vi "Shooter Solenoid Refnums fg.vi"(0 "Menu":T8, 1 "Shooter Solenoid DevRef":T4={"DevStatus"={"status"=FALSE, "code"=0, "source"=""}, "Solenoid Module"=enum."Solenoid Module 1", "Forward Solenoid Channel"=enum."Invalid", "Reverse Solenoid Channel"=enum."Invalid"}, 2 "Latch Solenoid DevRef":T4={"DevStatus"={"status"=FALSE, "code"=0, "source"=""}, "Solenoid Module"=enum."Solenoid Module 1", "Forward Solenoid Channel"=enum."Invalid", "Reverse Solenoid Channel"=enum."Invalid"}, 3 "Right Up DevRef":T1={"DevStatus"={"status"=FALSE, "code"=0, "source"=""}, "DIO Channel"=enum."Invalid", "Digital Module"=enum."Digital Module 1"}, 4 "Right Down DevRef":T1={"DevStatus"={"status"=FALSE, "code"=0, "source"=""}, "DIO Channel"=enum."Invalid", "Digital Module"=enum."Digital Module 1"}, 5 "Hold Sensor DevRef":T1={"DevStatus"={"status"=FALSE, "code"=0, "source"=""}, "DIO Channel"=enum."Invalid", "Digital Module"=enum."Digital Module 1"}, 8 "DevRef to Get":T7(ring)) -> (14 "Selected Solenoid":T4={"DevStatus"={"status"=FALSE, "code"=0, "source"=""}, "Solenoid Module"=enum."Solenoid Module 1", "Forward Solenoid Channel"=enum."Invalid", "Reverse Solenoid Channel"=enum."Invalid"}, 15 "Selected Sensor":T1)   [LabVIEW 2013]
uses:
  <vilib>/Rock Robotics/WPI/Solenoid/WPI_SolenoidDevRef.ctl
  <vilib>/Rock Robotics/SystemInterfaces/Typedef/FPGA_TypedefSolenoidModule.ctl
  <vilib>/Rock Robotics/WPI/Solenoid/WPI_SolenoidChannel.ctl
  <vilib>/Rock Robotics/WPI/DigitalInput/WPI_DigitalInputDevRef.ctl
  <vilib>/Rock Robotics/SystemInterfaces/DIO/FPGA_DIOChannel.ctl
  <vilib>/Rock Robotics/SystemInterfaces/Typedef/FPGA_TypedefDigitalModule.ctl
  typedefs/fg_typedef.ctl
panel:
  out "Hold Sensor DevRef":T1
  out "Right Down DevRef":T1
  out "Right Up DevRef":T1
  out "Latch Solenoid DevRef":T4={"DevStatus"={"status"=FALSE, "code"=0, "source"=""}, "Solenoid Module"=enum."Solenoid Module 1", "Forward Solenoid Channel"=enum."Invalid", "Reverse Solenoid Channel"=enum."Invalid"}
  out "Shooter Solenoid DevRef":T4={"DevStatus"={"status"=FALSE, "code"=0, "source"=""}, "Solenoid Module"=enum."Solenoid Module 1", "Forward Solenoid Channel"=enum."Invalid", "Reverse Solenoid Channel"=enum."Invalid"}
  # "A Functional Global that stores refnums for \ncommonly used devices \nso as to not need to get them repeatedly"
  # "Option to Select Also..."
  # "it is only set once"
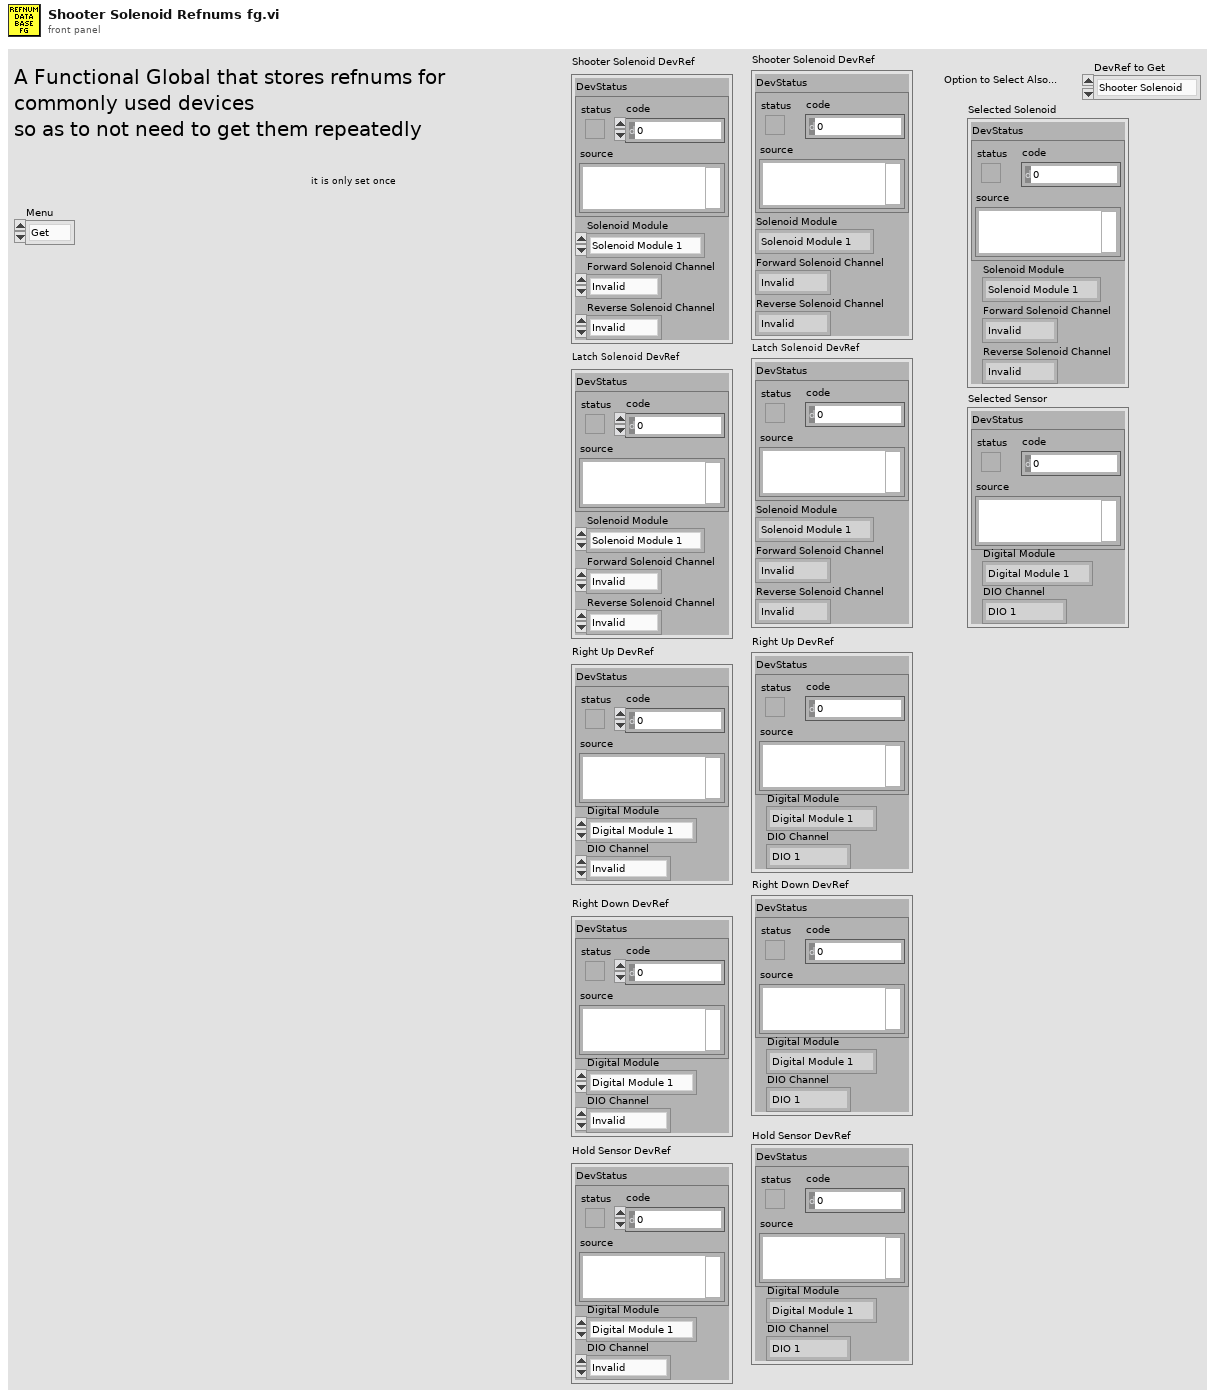
[diagram p1: front panel]
types:
  T1 = typedef "WPI_DigitalInputDevRef.ctl" = cluster{"DevStatus":errorcluster, "DIO Channel":T2, "Digital Module":T3}
  T2 = typedef "FPGA_DIOChannel.ctl" = enum8{"DIO 1", "DIO 2", "DIO 3", "DIO 4", "DIO 5", "DIO 6", "DIO 7", "DIO 8", "DIO 9", "DIO 10", "DIO 11", "DIO 12", "DIO 13", "DIO 14", "Invalid"}
  T3 = typedef "FPGA_TypedefDigitalModule.ctl" = enum16{"Digital Module 1", "Digital Module 2"}
  T4 = typedef "WPI_SolenoidDevRef.ctl" = cluster{"DevStatus":errorcluster, "Solenoid Module":T5, "Forward Solenoid Channel":T6, "Reverse Solenoid Channel":T6}
  T5 = typedef "FPGA_TypedefSolenoidModule.ctl" = enum16{"Solenoid Module 1", "Solenoid Module 2"}
  T6 = typedef "WPI_SolenoidChannel.ctl" = enum8{"Solenoid 1", "Solenoid 2", "Solenoid 3", "Solenoid 4", "Solenoid 5", "Solenoid 6", "Solenoid 7", "Solenoid 8", "Invalid"}
  T7 = enum16{"Shooter Solenoid", "Latch Solenoid", "Right Up Sensor", "Right Down Sensor", "Hold Sensor"}
  T8 = typedef "fg_typedef.ctl" = enum16{"Get", "Set"}
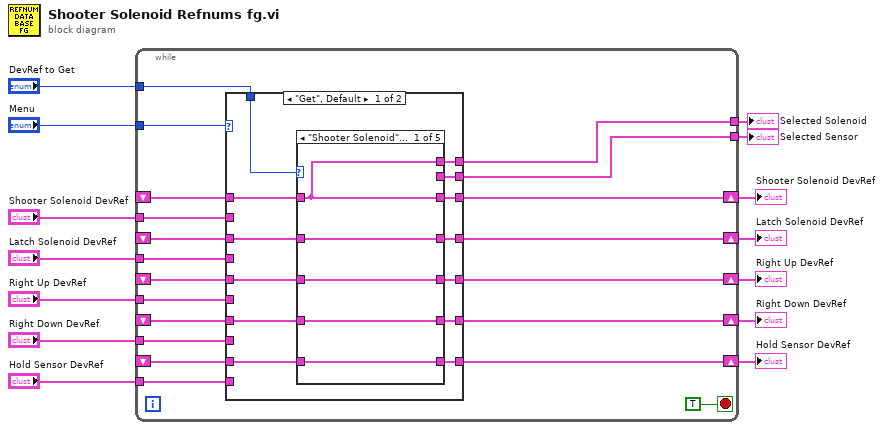
[diagram p0: block diagram]
diagram:
  n1 = while {
    shift-right: [w28] -> w14
    shift-left: _ -> [w33]
    shift-right: [w27] -> w13
    shift-left: _ -> [w32]
    shift-right: [w26] -> w12
    shift-left: _ -> [w30]
    shift-right: [w25] -> w11
    shift-left: _ -> [w29]
    tunnel: "Menu" -> [w31]
    tunnel: "Shooter Solenoid DevRef" -> [w24]
    tunnel: "Latch Solenoid DevRef" -> [w23]
    tunnel: "Right Up DevRef" -> [w22]
    tunnel: "Right Down DevRef" -> [w21]
    shift-right: [w18] -> w4
    shift-left: _ -> [w19]
    tunnel: "Hold Sensor DevRef" -> [w20]
    tunnel: "DevRef to Get" -> [w17]
    tunnel: [w16] -> w2
    tunnel: [w15] -> w1
    stop <- TRUE stop-if-true
    n2 = case shown="\"Get\", Default" w31 {
      tunnel: w33 -> [w46 _]
      tunnel: w32 -> [w45 _]
      tunnel: w30 -> [w44 _]
      tunnel: w29 -> [w43 _]
      tunnel: [w35 w77] -> w28
      tunnel: [w36 w76] -> w27
      tunnel: [w37 w75] -> w26
      tunnel: [w38 w74] -> w25
      tunnel: w24 -> [_ w77]
      tunnel: w23 -> [_ w76]
      tunnel: w22 -> [_ w75]
      tunnel: w21 -> [_ w74]
      tunnel: w20 -> [_ w73]
      tunnel: w19 -> [w42 _]
      tunnel: [w39 w73] -> w18
      tunnel: w17 -> [w47 _]
      tunnel: [w41 _] -> w16
      tunnel: [w40 _] -> w15
      frame "Get", Default {
        n3 = case shown="\"Shooter Solenoid\", Default" w47 {
          tunnel: w46 -> [w48 w57 w62 w67 w72]
          tunnel: w45 -> [w49 w56 w61 w66 w71]
          tunnel: w44 -> [w50 w55 w60 w65 w70]
          tunnel: w43 -> [w51 w54 w59 w64 w69]
          tunnel: w42 -> [w52 w53 w58 w63 w68]
          tunnel: [w48 w56 _ _ _] -> w41
          tunnel: [_ _ w60 w64 w68] -> w40
          tunnel: [w52 w53 w58 w63 w68] -> w39
          tunnel: [w51 w54 w59 w64 w69] -> w38
          tunnel: [w50 w55 w60 w65 w70] -> w37
          tunnel: [w49 w56 w61 w66 w71] -> w36
          tunnel: [w48 w57 w62 w67 w72] -> w35
          frame "Shooter Solenoid", Default {
          }
          frame "Latch Solenoid" {
          }
          frame "Right Up Sensor" {
          }
          frame "Right Down Sensor" {
          }
          frame "Hold Sensor" {
          }
        }
      }
      frame "Set" {
      }
    }
  }
  "Shooter Solenoid DevRef" <- w14
  "Latch Solenoid DevRef" <- w13
  "Right Up DevRef" <- w12
  "Right Down DevRef" <- w11
  "Hold Sensor DevRef" <- w4
  "Selected Solenoid" <- w2
  "Selected Sensor" <- w1
